vi "4_detected.vi"(0 "4-bit pixmap":u8[][](array[numeric]), 1 "moving Log(Row, Col.)":i32[][](array[numeric])) -> (2 "4 detected":bool, 3 "tapN":i32)   [LabVIEW 2016]
panel:
  out "root(Row, point)":i32[][](array[numeric])
  # "3でOUTにする理由：93 (IMG6145.PNG)"
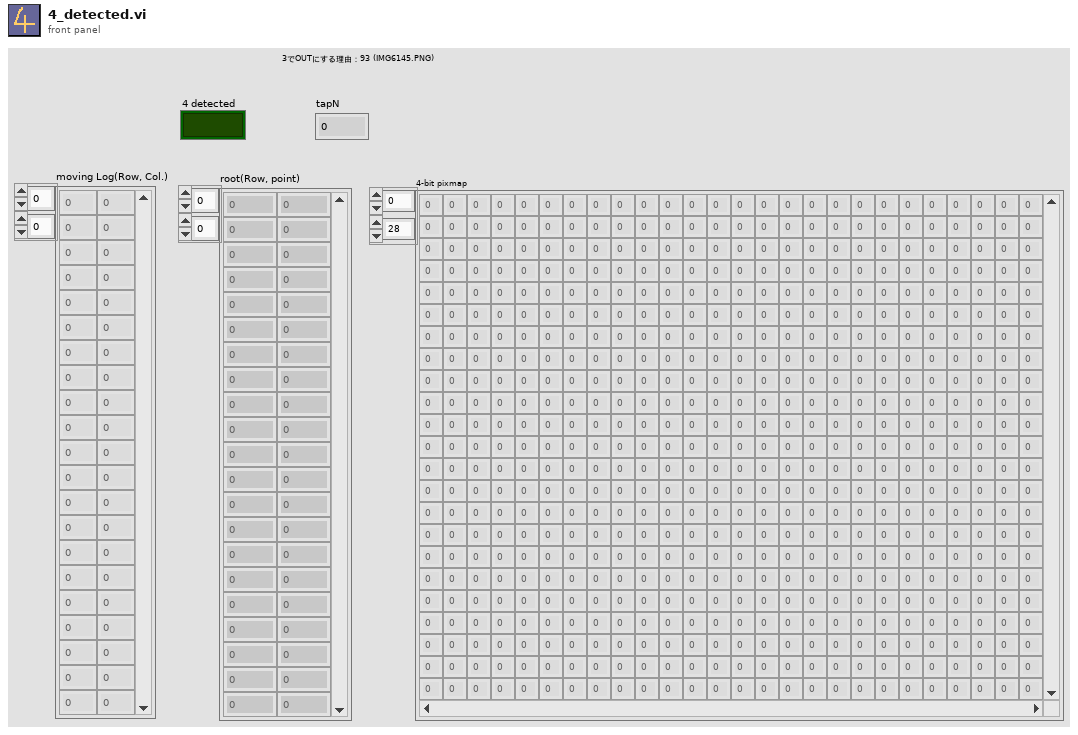
[diagram p1: front panel]
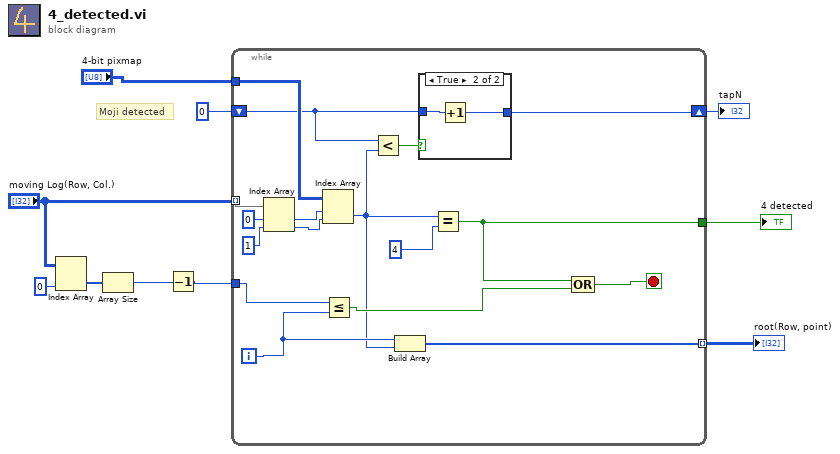
[diagram p0: block diagram]
diagram:
  # "Moji detected"
  n1 = Index Array(array="moving Log(Row, Col.)", index (col)=0 ("無効な指標 （列）")) -> (element=w7:i32[])  [unwired: 1 in]
  n2 = Array Size(array=w7) -> (size(s)=w4:i32)
  n3 = Decrement(x=w4) -> (x-1=w3:i32)
  n4 = while {
    tunnel: "moving Log(Row, Col.)" -> [w27] mode=indexing
    tunnel: "4-bit pixmap" -> [w24]
    tunnel: w3 -> [w20]
    tunnel: [w16] -> w5
    shift-right: [w15] -> w1
    shift-left: 0 ("指標") -> [w18]
    tunnel: [w11] -> w2 mode=indexing
    i -> [w13]
    stop <- w14 stop-if-true
    n5 = Index Array(array=w27, index #1=0 ("指標"), index #2=1 ("指標")) -> (element #1=w23:i32, element #2=w22:i32)
    n6 = Index Array(array=w24, index (row)=w23, index (col)=w22) -> (element=w12:u8)
    n7 = Less Or Equal?(x=w20, y=w13) -> (x <= y?=w17:bool)
    n8 = Less?(x=w18, y=w12) -> (x < y?=w19:bool)
    n9 = Build Array(w13, w12) -> (w11:i32[])
    n10 = case shown="True" w19 {
      tunnel: w18 -> [w28 w30]
      tunnel: [w28 w29] -> w15
      frame False {
      }
      frame True {
        n11 = Increment(x=w30) -> (x+1=w29:i32)
      }
    }
    n12 = Equal?(x=w12, y=4) -> (x = y?=w16:bool)
    n13 = Compound Arithmetic op=OR ("複合演算")(w16, w17) -> (w14:bool)
  }
  "4 detected" <- w5
  "root(Row, point)" <- w2
  "tapN" <- w1
